vi "S8300E_SetVoltage_CriteriaTOOL.vi"() -> ()   [LabVIEW 2011]
panel:
  in  "Tab Control":enum32{"Page 1", "Page 2"}(tab)
  in  "P1V0_PCH High Limit  Voltage":dbl format="%#.6f"
  in  "P1V0_PCH Lower Limit Voltage":dbl format="%#.6f"
  out "TestPoint_Name 6":string="TP46"
  in  "PVCCIO   High Limit  Voltage":dbl format="%#.6f"
  in  "PVCCIO Lower Limit  Voltage":dbl format="%#.6f"
  out "TestPoint_Name 4":string="TP46"
  in  "P1V8  High Limit  Voltage":dbl format="%#.6f"
  in  "P1V8 Lower Limit  Voltage":dbl format="%#.6f"
  out "TestPoint_Name 3":string="TP46"
  in  "P3V3  High Voltage":dbl format="%#.6f"
  in  "P3V3  Lower Voltage":dbl format="%#.6f"
  out "TestPoint_Name 2":string="TP46"
  in  "P5V High Limit Voltage":dbl format="%#.6f"
  in  "P5V Lower Limit Voltage":dbl format="%#.6f"
  out "TestPoint_Name":string="TP46"
  out "TestPoint_Name 7":string="TP46"
  in  "PVCCSA Lower Limit Voltage":dbl format="%#.6f"
  in  "PVCCSA High Limit  Voltage":dbl format="%#.6f"
  out "TestPoint_Name 8":string="TP46"
  in  "H-P1V5 Lower Limit Voltage":dbl format="%#.6f"
  in  "H-P1V5  High Limit  Voltage":dbl format="%#.6f"
  out "TestPoint_Name 9":string="TP46"
  in  "H-P0V75 Lower Limit Voltage":dbl format="%#.6f"
  in  "H-P0V75 High Limit  Voltage":dbl format="%#.6f"
  out "TestPoint_Name 10":string="TP46"
  in  "PVCCPLL Lower Limit Voltage":dbl format="%#.6f"
  in  "PVCCPLL High Limit  Voltage":dbl format="%#.6f"
  out "TestPoint_Name 11":string="TP46"
  in  "P3V3_S0  Lower Limit Voltage":dbl format="%#.6f"
  in  "P3V3_S0  High Limit  Voltage":dbl format="%#.6f"
  out "TestPoint_Name 12":string="TP46"
  in  "P1V05_PCH Lower Limit Voltage":dbl format="%#.6f"
  in  "P1V05_PCH High Limit  Voltage":dbl format="%#.6f"
  out "TestPoint_Name 13":string="TP46"
  in  "P1V5_PCH Lower Limit Voltage":dbl format="%#.6f"
  in  "P1V5_PCH High Limit  Voltage":dbl format="%#.6f"
  out "TestPoint_Name 14":string="TP46"
  in  "P1V8_PCH Lower Limit Voltage":dbl format="%#.6f"
  in  "P1V8_PCH High Limit  Voltage":dbl format="%#.6f"
  out "TestPoint_Name 15":string="TP46"
  in  "P3V3_PCH Lower Limit Voltage":dbl format="%#.6f"
  in  "P3V3_PCH High Limit  Voltage":dbl format="%#.6f"
  out "TestPoint_Name 16":string="TP46"
  in  "L-P1V5 Lower Limit Voltage":dbl format="%#.6f"
  in  "L-P1V5  High Limit  Voltage":dbl format="%#.6f"
  out "TestPoint_Name 17":string="TP46"
  in  "L-P0V75 Lower Limit Voltage":dbl format="%#.6f"
  in  "L-P0V75  High Limit  Voltage":dbl format="%#.6f"
  out "DatalogType":T1(array[cluster]) {"Lower Limit Voltage" format="%#.6f"; "High Limit Voltage" format="%#.6f"}
  in  "儲存離開":bool
  # "2014-11-21"
  # "S8300E Test Point Voltage Criteria Setting\nS8300E 各測點 電壓  設定"
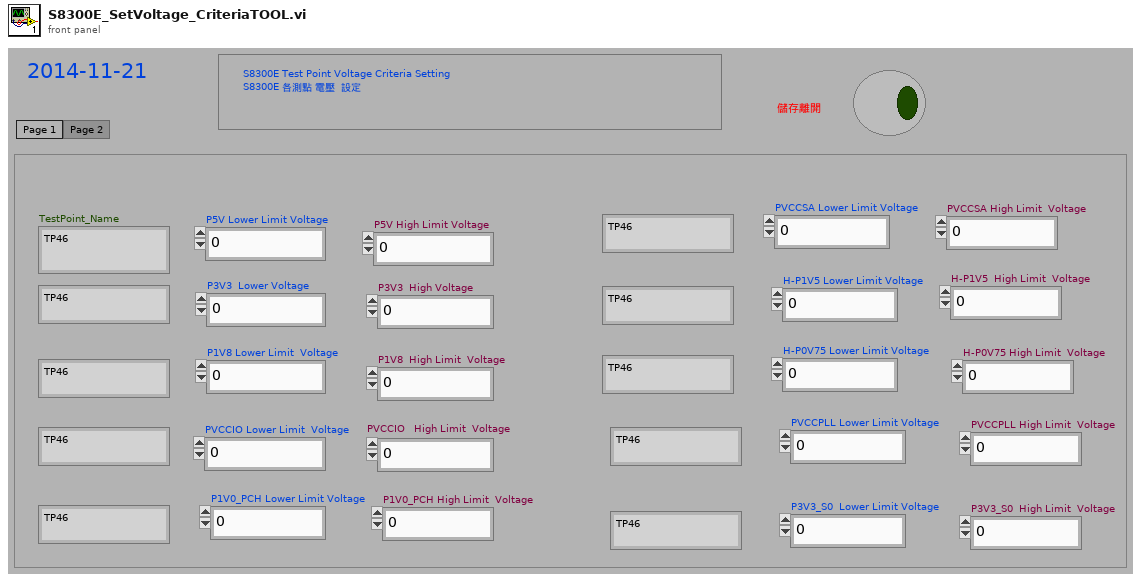
[diagram p1: front panel]
types:
  T1 = cluster{"TestPoint_Name":string, "Lower Limit Voltage":dbl, "High Limit Voltage":dbl, cluster{"Relay3 Name":string, "Relay3H/L":bool}[], "Measure Ai name":string}[]
  T2 = enum16{"open", "replace", "create", "open or create", "replace or create", "replace or create with confirmation"}
  T3 = cluster{"TestPoint_Name":string, "Lower Limit Voltage":dbl, "High Limit Voltage":dbl, cluster{"Relay3 Name":string, "Relay3H/L":bool}[], "Measure Ai name":string}
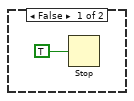
[diagram p2: hidden frame]
diagram:
  n1 = flat-sequence {
    tunnel: [w66] -> w1
    tunnel: w1 -> [w259]
    frame #0 {
      n2 = call "SUB_Password_keyin.vi"() -> ("Pass?"=w2:bool)  [unwired: 3 in]
      n3 = case shown="True" w2 {
        frame False {
          n4 = Stop(stop? (T)=TRUE) -> ()
        }
        frame True {
        }
      }
    }
    frame #1 {
      n5 = call "SUB_SearchFile_inFolder.vi"("Search Filename in Folder"="S8300E_TP_Voltage.dat" ("name or relative path")) -> ("File Existing True/Flase"=w4:bool)  [unwired: 1 in]
      n6 = case shown="True" w4 {
        frame False {
        }
        frame True {
          n7 = flat-sequence {
            frame #0 {
              n8 = call "SUB_RunTime_FilePath.vi"() -> ("stripped path"=w56:path)  [unwired: 3 in]
              n9 = Build Path(base path=w56, name or relative path="S8300E_TP_Voltage.dat") -> (appended path=w61:path)
              n10 = local read "DatalogType"() -> (w55:T1)
              n11 = Open/Create/Replace Datalog(5:w55, 9:enum16{"read/write", "read-only", "write-only"}."read-only" ("access (0:read/write)"), 10:T2."open" ("operation (0:open)"), 11:w61) -> (0:w58:errorcluster, 3:w57:refnum<k1>)  [unwired: 2 in, 1 out]
              n12 = Read Datalog(4:w58, 7:w57) -> (0:w60:errorcluster, 2:w54:T1, 3:w59:refnum<k1>)  [unwired: 1 in]
              n13 = Close File(refnum=w59, error in=w60) -> ()  [unwired: 2 out]
              n14 = Index Array(array=w54) -> (element #1=w53:T3, element #2=w50:T3, element #3=w47:T3, element #4=w44:T3, element #5=w41:T3, element #6=w38:T3, element #7=w35:T3, element #8=w32:T3, element #9=w29:T3, element #10=w26:T3, element #11=w23:T3, element #12=w20:T3, element #13=w17:T3, element #14=w14:T3, element #15=w11:T3, element #16=w10:T3)  [unwired: 16 in]
              n15 = Unbundle By Name(w10) -> ("Lower Limit Voltage"=w7:dbl, "High Limit Voltage"=w6:dbl)
              n16 = Unbundle By Name(w11) -> ("Lower Limit Voltage"=w9:dbl, "High Limit Voltage"=w8:dbl)
              n17 = Unbundle By Name(w23) -> ("Lower Limit Voltage"=w22:dbl, "High Limit Voltage"=w21:dbl)
              n18 = Unbundle By Name(w26) -> ("Lower Limit Voltage"=w25:dbl, "High Limit Voltage"=w24:dbl)
              n19 = Unbundle By Name(w20) -> ("Lower Limit Voltage"=w19:dbl, "High Limit Voltage"=w18:dbl)
              n20 = Unbundle By Name(w17) -> ("Lower Limit Voltage"=w16:dbl, "High Limit Voltage"=w15:dbl)
              n21 = Unbundle By Name(w29) -> ("Lower Limit Voltage"=w28:dbl, "High Limit Voltage"=w27:dbl)
              n22 = Unbundle By Name(w38) -> ("Lower Limit Voltage"=w37:dbl, "High Limit Voltage"=w36:dbl)
              n23 = Unbundle By Name(w53) -> ("Lower Limit Voltage"=w52:dbl, "High Limit Voltage"=w51:dbl)
              n24 = Unbundle By Name(w47) -> ("Lower Limit Voltage"=w46:dbl, "High Limit Voltage"=w45:dbl)
              n25 = Unbundle By Name(w50) -> ("Lower Limit Voltage"=w49:dbl, "High Limit Voltage"=w48:dbl)
              n26 = Unbundle By Name(w32) -> ("Lower Limit Voltage"=w31:dbl, "High Limit Voltage"=w30:dbl)
              n27 = Unbundle By Name(w41) -> ("Lower Limit Voltage"=w40:dbl, "High Limit Voltage"=w39:dbl)
              n28 = Unbundle By Name(w35) -> ("Lower Limit Voltage"=w34:dbl, "High Limit Voltage"=w33:dbl)
              n29 = Unbundle By Name(w14) -> ("Lower Limit Voltage"=w13:dbl, "High Limit Voltage"=w12:dbl)
              n30 = Unbundle By Name(w44) -> ("Lower Limit Voltage"=w43:dbl, "High Limit Voltage"=w42:dbl)
              n31 = local write "P1V05_PCH Lower Limit Voltage"(w22) -> ()
              n32 = local write "L-P0V75  High Limit  Voltage"(w6) -> ()
              n33 = local write "P3V3_S0  Lower Limit Voltage"(w25) -> ()
              n34 = local write "P3V3_S0  High Limit  Voltage"(w24) -> ()
              n35 = local write "L-P0V75 Lower Limit Voltage"(w7) -> ()
              n36 = local write "P1V0_PCH Lower Limit Voltage"(w40) -> ()
              n37 = local write "H-P1V5 Lower Limit Voltage"(w34) -> ()
              n38 = local write "L-P1V5 Lower Limit Voltage"(w9) -> ()
              n39 = local write "L-P1V5  High Limit  Voltage"(w8) -> ()
              n40 = local write "P1V05_PCH High Limit  Voltage"(w21) -> ()
              n41 = local write "P1V0_PCH High Limit  Voltage"(w39) -> ()
              n42 = local write "P5V Lower Limit Voltage"(w52) -> ()
              n43 = local write "PVCCSA Lower Limit Voltage"(w37) -> ()
              n44 = local write "H-P0V75 Lower Limit Voltage"(w31) -> ()
              n45 = local write "P1V8_PCH Lower Limit Voltage"(w16) -> ()
              n46 = local write "P1V8_PCH High Limit  Voltage"(w15) -> ()
              n47 = local write "H-P1V5  High Limit  Voltage"(w33) -> ()
              n48 = local write "P5V High Limit Voltage"(w51) -> ()
              n49 = local write "P1V5_PCH Lower Limit Voltage"(w19) -> ()
              n50 = local write "PVCCIO Lower Limit  Voltage"(w43) -> ()
              n51 = local write "H-P0V75 High Limit  Voltage"(w30) -> ()
              n52 = local write "PVCCSA High Limit  Voltage"(w36) -> ()
              n53 = local write "P1V8 Lower Limit  Voltage"(w46) -> ()
              n54 = local write "PVCCPLL High Limit  Voltage"(w27) -> ()
              n55 = local write "PVCCPLL Lower Limit Voltage"(w28) -> ()
              n56 = local write "P3V3_PCH Lower Limit Voltage"(w13) -> ()
              n57 = local write "P1V5_PCH High Limit  Voltage"(w18) -> ()
              n58 = local write "PVCCIO   High Limit  Voltage"(w42) -> ()
              n59 = local write "P1V8  High Limit  Voltage"(w45) -> ()
              n60 = local write "P3V3_PCH High Limit  Voltage"(w12) -> ()
              n61 = local write "P3V3  Lower Voltage"(w49) -> ()
              n62 = local write "P3V3  High Voltage"(w48) -> ()
            }
          }
        }
      }
    }
    frame #2 {
      n63 = invoke on="儲存離開" class="Bool (strict)" method="Reinit To Default"() -> ()  [unwired: 3 in, 3 out]
      n64 = property on="儲存離開" class="Bool (strict)"("Blinking"=TRUE) -> ()  [unwired: 2 in, 2 out]
    }
    frame #3 {
      n65 = while {
        tunnel: [w213] -> w66
        stop <- "儲存離開" stop-if-true
        w87 = FALSE
        w88 = ""
        w95 = "L-P0V75" ("TestPoint_Name")
        w97 = FALSE
        w98 = ""
        w104 = "L-P1V5" ("TestPoint_Name")
        w115 = FALSE
        w116 = ""
        w123 = " P3V3_PCH" ("TestPoint_Name")
        w125 = FALSE
        w126 = ""
        w133 = "P1V8_PCH" ("TestPoint_Name")
        w135 = FALSE
        w136 = ""
        w143 = "P1V5_PCH" ("TestPoint_Name")
        w145 = FALSE
        w146 = ""
        w153 = "P1V05_PCH" ("TestPoint_Name")
        w155 = FALSE
        w156 = ""
        w163 = "P3V3_S0" ("TestPoint_Name")
        w165 = FALSE
        w166 = ""
        w173 = "PVCCPLL" ("TestPoint_Name")
        w175 = FALSE
        w176 = ""
        w183 = "H-P0V75" ("TestPoint_Name")
        w185 = FALSE
        w186 = ""
        w193 = "H-P1V5" ("TestPoint_Name")
        w199 = FALSE
        w200 = ""
        w207 = "PVCCSA" ("TestPoint_Name")
        w219 = FALSE
        w220 = ""
        w221 = FALSE
        w222 = ""
        w197 = ""
        w225 = ""
        w211 = ""
        w234 = "P1V0_PCH" ("TestPoint_Name")
        w241 = "PVCCIO" ("TestPoint_Name")
        w223 = FALSE
        w247 = "P1V8" ("TestPoint_Name")
        w224 = FALSE
        w253 = "P3V3" ("TestPoint_Name")
        w226 = FALSE
        w258 = "P5V" ("TestPoint_Name")
        # "04"
        # "03"
        # "02"
        # "01"
        # "00"
        n66 = call "SUB_s8300E-TestPoint_Format.vi"("TestPoint_Name"=w123, "Lower Limit Voltage"="P3V3_PCH Lower Limit Voltage", "High Limit Voltage"="P3V3_PCH High Limit  Voltage", "Relay 1 Name"="2.0", "Relay1 H/L"=FALSE, "Relay 2 Name"="", "Relay2 H/L"=FALSE, "Relay3 Name"=w116, "Relay3H/L"=FALSE, "Measure Ai name"="./volt.sh 14", "Relay4 Name"=w116, "Relay4 H/L"=w115, "Relay5 Name"=w116, "Relay5 H/L"=w115) -> ("output cluster"=w105:T3)  [unwired: 13 in]
        n67 = call "SUB_s8300E-TestPoint_Format.vi"("TestPoint_Name"=w143, "Lower Limit Voltage"="P1V5_PCH Lower Limit Voltage", "High Limit Voltage"="P1V5_PCH High Limit  Voltage", "Relay 1 Name"="1.0", "Relay1 H/L"=FALSE, "Relay 2 Name"="", "Relay2 H/L"=FALSE, "Relay3 Name"=w136, "Relay3H/L"=FALSE, "Measure Ai name"="./volt.sh 12", "Relay4 Name"=w136, "Relay4 H/L"=w135, "Relay5 Name"=w136, "Relay5 H/L"=w135) -> ("output cluster"=w107:T3)  [unwired: 13 in]
        n68 = call "SUB_s8300E-TestPoint_Format.vi"("TestPoint_Name"=w133, "Lower Limit Voltage"="P1V8_PCH Lower Limit Voltage", "High Limit Voltage"="P1V8_PCH High Limit  Voltage", "Relay 1 Name"="1.0", "Relay1 H/L"=FALSE, "Relay 2 Name"="", "Relay2 H/L"=FALSE, "Relay3 Name"=w126, "Relay3H/L"=FALSE, "Measure Ai name"="./volt.sh 13", "Relay4 Name"=w126, "Relay4 H/L"=w125, "Relay5 Name"=w126, "Relay5 H/L"=w125) -> ("output cluster"=w106:T3)  [unwired: 13 in]
        n69 = call "SUB_s8300E-TestPoint_Format.vi"("TestPoint_Name"=w153, "Lower Limit Voltage"="P1V05_PCH Lower Limit Voltage", "High Limit Voltage"="P1V05_PCH High Limit  Voltage", "Relay 1 Name"="1.0", "Relay1 H/L"=FALSE, "Relay 2 Name"="", "Relay2 H/L"=FALSE, "Relay3 Name"=w146, "Relay3H/L"=FALSE, "Measure Ai name"="./volt.sh 11", "Relay4 Name"=w146, "Relay4 H/L"=w145, "Relay5 Name"=w146, "Relay5 H/L"=w145) -> ("output cluster"=w108:T3)  [unwired: 13 in]
        n70 = call "SUB_s8300E-TestPoint_Format.vi"("TestPoint_Name"=w163, "Lower Limit Voltage"="P3V3_S0  Lower Limit Voltage", "High Limit Voltage"="P3V3_S0  High Limit  Voltage", "Relay 1 Name"="2.0", "Relay1 H/L"=FALSE, "Relay 2 Name"="", "Relay2 H/L"=FALSE, "Relay3 Name"=w156, "Relay3H/L"=FALSE, "Measure Ai name"="./volt.sh 10", "Relay4 Name"=w156, "Relay4 H/L"=w155, "Relay5 Name"=w156, "Relay5 H/L"=w155) -> ("output cluster"=w109:T3)  [unwired: 13 in]
        n71 = call "SUB_s8300E-TestPoint_Format.vi"("TestPoint_Name"=w183, "Lower Limit Voltage"="H-P0V75 Lower Limit Voltage", "High Limit Voltage"="H-P0V75 High Limit  Voltage", "Relay 1 Name"="1.0", "Relay1 H/L"=FALSE, "Relay 2 Name"="", "Relay2 H/L"=FALSE, "Relay3 Name"=w176, "Relay3H/L"=FALSE, "Measure Ai name"="./volt.sh 8", "Relay4 Name"=w176, "Relay4 H/L"=w175, "Relay5 Name"=w176, "Relay5 H/L"=w175) -> ("output cluster"=w111:T3)  [unwired: 13 in]
        n72 = call "SUB_s8300E-TestPoint_Format.vi"("TestPoint_Name"=w234, "Lower Limit Voltage"="P1V0_PCH Lower Limit Voltage", "High Limit Voltage"="P1V0_PCH High Limit  Voltage", "Relay 1 Name"="1.0", "Relay1 H/L"=FALSE, "Relay 2 Name"="", "Relay2 H/L"=FALSE, "Relay3 Name"=w220, "Relay3H/L"=FALSE, "Measure Ai name"="./volt.sh 5", "Relay4 Name"=w220, "Relay4 H/L"=w219, "Relay5 Name"=w220, "Relay5 H/L"=w219) -> ("output cluster"=w214:T3)  [unwired: 13 in]
        n73 = call "SUB_s8300E-TestPoint_Format.vi"("TestPoint_Name"=w95, "Lower Limit Voltage"="L-P0V75 Lower Limit Voltage", "High Limit Voltage"="L-P0V75  High Limit  Voltage", "Relay 1 Name"="1.0", "Relay1 H/L"=FALSE, "Relay 2 Name"="", "Relay2 H/L"=FALSE, "Relay3 Name"=w88, "Relay3H/L"=FALSE, "Measure Ai name"="./volt.sh 8", "Relay4 Name"=w88, "Relay4 H/L"=w87, "Relay5 Name"=w88, "Relay5 H/L"=w87) -> ("output cluster"=w83:T3)  [unwired: 13 in]
        n74 = call "SUB_s8300E-TestPoint_Format.vi"("TestPoint_Name"=w173, "Lower Limit Voltage"="PVCCPLL Lower Limit Voltage", "High Limit Voltage"="PVCCPLL High Limit  Voltage", "Relay 1 Name"="1.0", "Relay1 H/L"=FALSE, "Relay 2 Name"="", "Relay2 H/L"=FALSE, "Relay3 Name"=w166, "Relay3H/L"=FALSE, "Measure Ai name"="./volt.sh 9", "Relay4 Name"=w166, "Relay4 H/L"=w165, "Relay5 Name"=w166, "Relay5 H/L"=w165) -> ("output cluster"=w110:T3)  [unwired: 13 in]
        n75 = call "SUB_s8300E-TestPoint_Format.vi"("TestPoint_Name"=w207, "Lower Limit Voltage"="PVCCSA Lower Limit Voltage", "High Limit Voltage"="PVCCSA High Limit  Voltage", "Relay 1 Name"="1.0", "Relay1 H/L"=FALSE, "Relay 2 Name"="", "Relay2 H/L"=FALSE, "Relay3 Name"=w200, "Relay3H/L"=FALSE, "Measure Ai name"="./volt.sh 6", "Relay4 Name"=w200, "Relay4 H/L"=w199, "Relay5 Name"=w200, "Relay5 H/L"=w199) -> ("output cluster"=w113:T3)  [unwired: 13 in]
        n76 = call "SUB_s8300E-TestPoint_Format.vi"("TestPoint_Name"=w193, "Lower Limit Voltage"="H-P1V5 Lower Limit Voltage", "High Limit Voltage"="H-P1V5  High Limit  Voltage", "Relay 1 Name"="1.0", "Relay1 H/L"=FALSE, "Relay 2 Name"="", "Relay2 H/L"=FALSE, "Relay3 Name"=w186, "Relay3H/L"=FALSE, "Measure Ai name"="./volt.sh 7", "Relay4 Name"=w186, "Relay4 H/L"=w185, "Relay5 Name"=w186, "Relay5 H/L"=w185) -> ("output cluster"=w112:T3)  [unwired: 13 in]
        n77 = call "SUB_s8300E-TestPoint_Format.vi"("TestPoint_Name"=w104, "Lower Limit Voltage"="L-P1V5 Lower Limit Voltage", "High Limit Voltage"="L-P1V5  High Limit  Voltage", "Relay 1 Name"="1.0", "Relay1 H/L"=FALSE, "Relay 2 Name"="", "Relay2 H/L"=FALSE, "Relay3 Name"=w98, "Relay3H/L"=FALSE, "Measure Ai name"="./volt.sh 7", "Relay4 Name"=w98, "Relay4 H/L"=w97, "Relay5 Name"=w98, "Relay5 H/L"=w97) -> ("output cluster"=w84:T3)  [unwired: 13 in]
        n78 = call "SUB_s8300E-TestPoint_Format.vi"("TestPoint_Name"=w241, "Lower Limit Voltage"="PVCCIO Lower Limit  Voltage", "High Limit Voltage"="PVCCIO   High Limit  Voltage", "Relay 1 Name"="1.0", "Relay1 H/L"=FALSE, "Relay 2 Name"="", "Relay2 H/L"=FALSE, "Relay3 Name"=w222, "Relay3H/L"=FALSE, "Measure Ai name"="./volt.sh 4", "Relay4 Name"=w222, "Relay4 H/L"=w221, "Relay5 Name"=w222, "Relay5 H/L"=w221) -> ("output cluster"=w215:T3)  [unwired: 13 in]
        n79 = call "SUB_s8300E-TestPoint_Format.vi"("TestPoint_Name"=w247, "Lower Limit Voltage"="P1V8 Lower Limit  Voltage", "High Limit Voltage"="P1V8  High Limit  Voltage", "Relay 1 Name"="1.0", "Relay1 H/L"=FALSE, "Relay 2 Name"="", "Relay2 H/L"=FALSE, "Relay3 Name"=w197, "Relay3H/L"=w223, "Measure Ai name"="./volt.sh 3", "Relay4 Name"=w197, "Relay4 H/L"=w223, "Relay5 Name"=w197, "Relay5 H/L"=w223) -> ("output cluster"=w216:T3)  [unwired: 13 in]
        n80 = call "SUB_s8300E-TestPoint_Format.vi"("TestPoint_Name"=w253, "Lower Limit Voltage"="P3V3  Lower Voltage", "High Limit Voltage"="P3V3  High Voltage", "Relay 1 Name"="2.0", "Relay1 H/L"=FALSE, "Relay 2 Name"="", "Relay2 H/L"=FALSE, "Relay3 Name"=w225, "Relay3H/L"=w224, "Measure Ai name"="./volt.sh 2", "Relay4 Name"=w225, "Relay4 H/L"=w224, "Relay5 Name"=w225, "Relay5 H/L"=w224) -> ("output cluster"=w217:T3)  [unwired: 13 in]
        n81 = call "SUB_s8300E-TestPoint_Format.vi"("TestPoint_Name"=w258, "Lower Limit Voltage"="P5V Lower Limit Voltage", "High Limit Voltage"="P5V High Limit Voltage", "Relay 1 Name"="3.127659574", "Relay1 H/L"=FALSE, "Relay 2 Name"="", "Relay2 H/L"=FALSE, "Relay3 Name"=w211, "Relay3H/L"=w226, "Measure Ai name"="./volt.sh 1", "Relay4 Name"=w211, "Relay4 H/L"=w226, "Relay5 Name"=w211, "Relay5 H/L"=w226) -> ("output cluster"=w218:T3)  [unwired: 13 in]
        n82 = Build Array "Build Array"(w218, w217, w216, w215, w214, w113, w112, w111, w110, w109, w108, w107, w106, w105, w84, w83) -> (w213:T1)
        n83 = Wait (ms)(milliseconds to wait=u32 100) -> ()  [unwired: 1 out]
        "TestPoint_Name" <- w258
        "TestPoint_Name 2" <- w253
        "TestPoint_Name 3" <- w247
        "TestPoint_Name 4" <- w241
        "TestPoint_Name 6" <- w234
        "TestPoint_Name 7" <- w207
        "TestPoint_Name 8" <- w193
        "TestPoint_Name 9" <- w183
        "TestPoint_Name 10" <- w173
        "TestPoint_Name 11" <- w163
        "TestPoint_Name 12" <- w153
        "TestPoint_Name 13" <- w143
        "TestPoint_Name 14" <- w133
        "TestPoint_Name 15" <- w123
        "TestPoint_Name 16" <- w104
        "TestPoint_Name 17" <- w95
      }
    }
    frame #4 {
      n84 = call "SUB_RunTime_FilePath.vi"() -> ("stripped path"=w261:path)  [unwired: 3 in]
      n85 = Build Path(base path=w261, name or relative path="S8300E_TP_Voltage.dat") -> (appended path=w262:path)
      n86 = Open/Create/Replace Datalog(5:w259, 9:enum16{"read/write", "read-only", "write-only"}."read/write" ("access (0:read/write)"), 10:T2."replace or create" ("operation (0:open)"), 11:w262) -> (0:w267:errorcluster, 3:w260:refnum<k1>)  [unwired: 2 in, 1 out]
      n87 = Write Datalog(4:w267, 6:w259, 7:w260) -> (0:w265:errorcluster, 3:w266:refnum<k1>)
      n88 = Close File(refnum=w266, error in=w265) -> ()  [unwired: 2 out]
      "DatalogType" <- w259
    }
    frame #5 {
      n89 = Quit LabVIEW(quit? (T)=FALSE) -> ()
    }
  }
